vi "Read Gantry Controller AUTOMATION1.vi"(8 "error in (no error)":errorcluster, 11 "Gantry in":refnum<class "Gantry.lvclass">) -> (0 "error out":errorcluster, 2 "Controller AUTOMATION1":refnum<k24>, 3 "Gantry out":refnum<class "Gantry.lvclass">)   [LabVIEW 2026, in "Gantry.lvclass"]
uses:
  Gantry.lvclass
  <instrlib>/Aerotech Automation1/Aerotech.Automation1.DotNet.dll
  Gantry.lvclass/Gantry.ctl
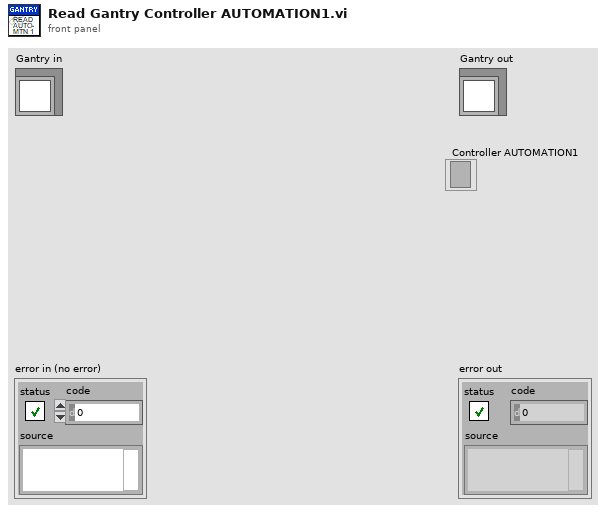
[diagram p1: front panel]
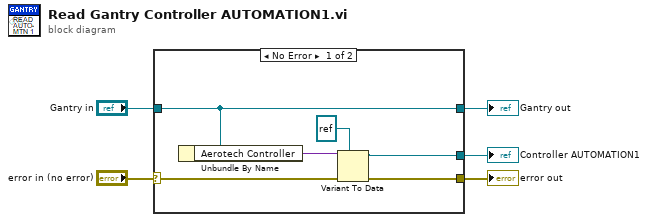
[diagram p0: block diagram]
diagram:
  n1 = case shown="No Error" "error in (no error)" {
    selector: "error in (no error)" -> [w9 w13]
    tunnel: [w8 w13] -> w4
    tunnel: [w11 w12] -> w2
    tunnel: "Gantry in" -> [w11 w12]
    tunnel: [w6 _] -> w1
    frame No Error {
      n2 = Unbundle By Name(w11) -> ("Aerotech Controller"=w10:variant)
      n3 = Variant To Data(error in=w9, type=refnum<k24> refnum ("Controller Refnum out"), Variant=w10) -> (data=w6:refnum<k24>, error out=w8:errorcluster)
    }
    frame Error {
    }
  }
  "error out" <- w4
  "Gantry out" <- w2
  "Controller AUTOMATION1" <- w1
